vi "Keithley2612b_IV_vg_vd_reverse_sweeps_modified.vi"(3 "Error Query (False)":bool, 4 "Current Limit":dbl=1.0, 7 "Source Function (Current)":enum32{"Current", "Voltage"}(ring)=enum."Voltage", 8 "error in (no error)":errorcluster, 9 "Channel (Channel A)":T1, 10 "Node (0-64)":i8 min=0 max=64 step=1, 11 "VISA resource name":refnum<visa-resource-name>="Keithley_2612B") -> (0 "error out":errorcluster)   [LabVIEW 2016]
doc: "This example shows how to configure the source and take a measurement."
uses:
  <instrlib>/Keithley 2600 Series/Public/Channel.ctl
  <vilib>/express/express shared/transition.llb/Dynamic To Waveform Array.vi
  <vilib>/express/express signal manip/GetorSetDDTAttributes/Set DDT Attributes/SetT0.vi
  <vilib>/express/express shared/transition.llb/Waveform Array To Dynamic.vi
  <vilib>/express/express signal manip/GetorSetDDTAttributes/Set DDT Attributes/Set DDT Properties.xnode
  <instrlib>/Keithley 2600 Series/Keithley 2600 Series.lvlib
panel:
  out "Number for Vg":dbl
  out "Step Size ref":dbl
  out "XY Graph":cluster{dbl[], dbl[]}[](graph)
  out "Current Number":dbl
  in  "Reverse Sweep":bool
  in  "Current Limit 2":dbl=1.0
  in  "Source Function (Current) 2":enum32{"Current", "Voltage"}(ring)=enum."Voltage"
  in  "Channel (Channel A) 2":T1=enum."Channel B"
  out "Current Output 2":string
  in  "Delay (s) 2":dbl
  in  "Step Size 2":dbl=0.02
  in  "End Voltage 2":dbl=0.8
  in  "Start Voltage 2":dbl=-0.5
  out "Voltage Output 2":string
  out "Current Number Past 2":dbl
  out "Current Number Past":dbl
  out "Voltage Output":string
  out "Current Output":string
  in  "Delay (s)":dbl
  in  "Step Size":dbl=0.1
  in  "End Voltage":dbl=1.0
  in  "Start Voltage":dbl
  # "Gate Voltage"
  # "Drain Voltage"
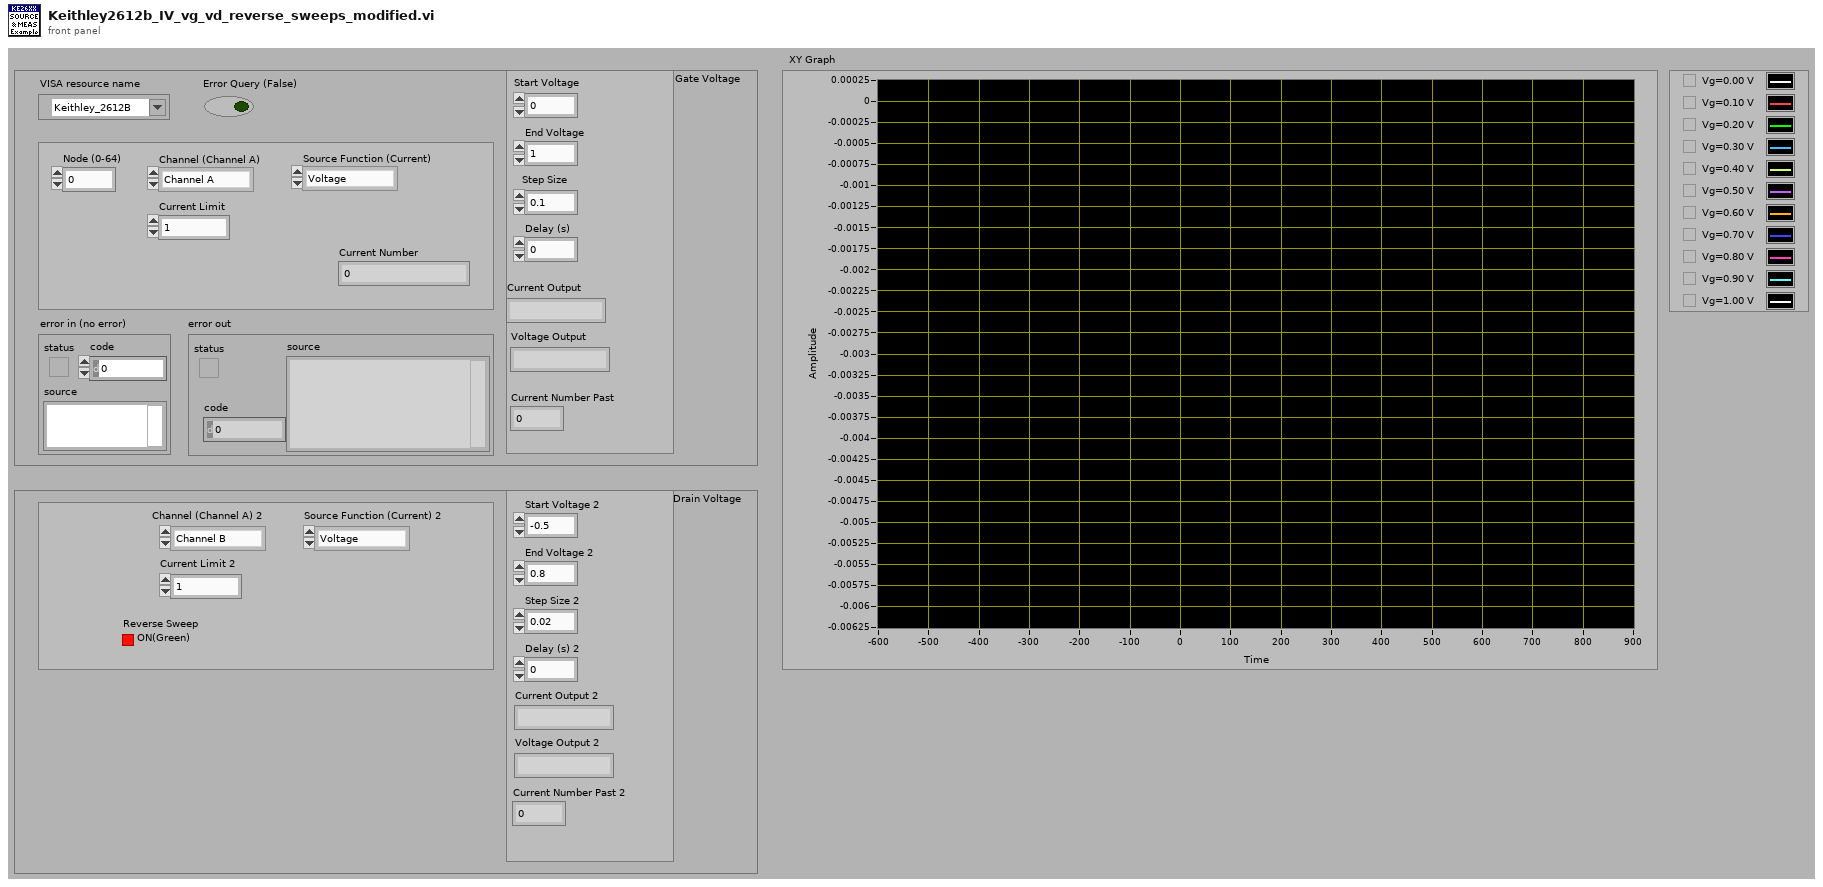
[diagram p1: front panel]
types:
  T1 = typedef "Keithley 2600 Series.lvlib/Channel.ctl" = enum32{"Channel A", "Channel B"}
  T2 = typedef "NI_Matrix.lvlib/RealMatrix.ctl" = dbl[][]
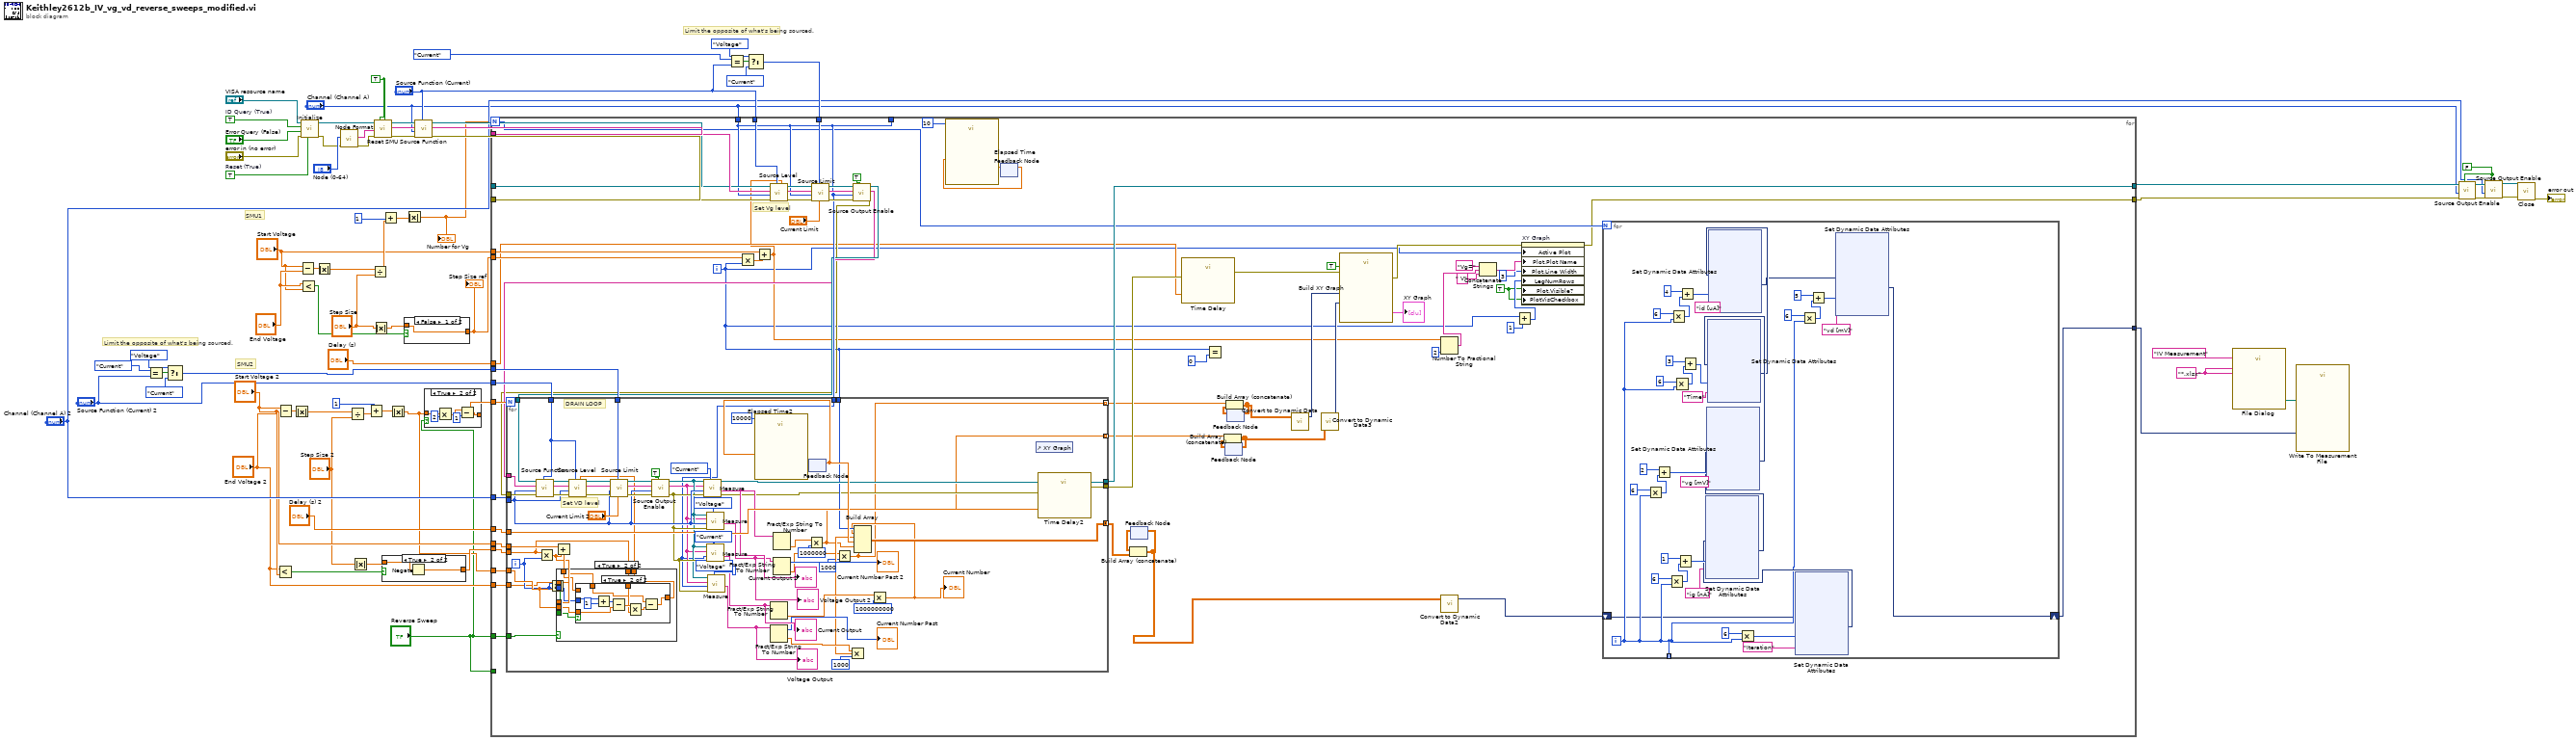
[diagram p0: block diagram]
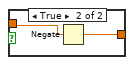
[diagram p3: hidden frame]
diagram:
  w29 = "*.xlsx"
  w40 = TRUE
  w24 = FALSE ("Output (Off)")
  w68 = TRUE  # Reset (True)
  w71 = TRUE  # ID Query (True)
  # "SMU2"
  # "SMU1"
  # "Limit the opposite of what's being sourced."
  # "Limit the opposite of what's being sourced."
  n1 = Equal?(x=enum32{"Current", "Voltage"}."Current", y="Source Function (Current) 2") -> (x = y?=w46:bool)
  n2 = Select(t=enum32{"Current", "Voltage"}."Voltage" ("x"), s=w46, f=enum32{"Current", "Voltage"}."Current") -> (s? t:f=w30:enum32{"Current", "Voltage"})
  n3 = Less?(x="End Voltage 2", y="Start Voltage 2") -> (x < y?=w20:bool)
  n4 = Subtract(x="Start Voltage 2", y="End Voltage 2") -> (x-y=w36:dbl)
  n5 = Absolute Value(x=w36) -> (abs(x)=w35:dbl)
  n6 = Subtract(x="Start Voltage", y="End Voltage") -> (x-y=w52:dbl)
  n7 = Less?(x="End Voltage", y="Start Voltage") -> (x < y?=w17:bool)
  n8 = call <instrlib>:"Initialize.vi"("Reset (True)"=w68, "error in (no error)"="error in (no error)", "Error Query (False)"="Error Query (False)", "ID Query (True)"=w71, "VISA resource name"="VISA resource name") -> ("error out"=w48:errorcluster, "VISA resource name out"=w41:refnum<visa-resource-name>)  [unwired: 1 in, 4 out]
  n9 = Absolute Value(x=w52) -> (abs(x)=w51:dbl)
  n10 = call <instrlib>:"Node Format.vi"("error in"=w48, "Node (0-64)"="Node (0-64)") -> ("error out"=w64:errorcluster, "Formatted Node"=w65:string)  [unwired: 8 out]
  n11 = Divide(x=w35, y="Step Size 2") -> (x/y=w33:dbl)
  n12 = Absolute Value(x="Step Size 2") -> (abs(x)=w14:dbl)
  n13 = Add(x=1, y=w33) -> (x+y=w12:dbl)
  n14 = Divide(x=w51, y="Step Size") -> (x/y=w49:dbl)
  n15 = Absolute Value(x="Step Size") -> (abs(x)=w8:dbl)
  n16 = call <instrlib>:"Reset SMU.vi"("SMU B (No)"=w40, "SMU A (No)"=w40, "error in (no error)"=w64, "Node In"=w65, "VISA resource name"=w41) -> ("error out"=w39:errorcluster, "Node Out"=w37:string, "VISA resource name out"=w38:refnum<visa-resource-name>)  [unwired: 4 out]
  n17 = Add(x=1, y=w49) -> (x+y=w11:dbl)
  n18 = case shown="True" w20 {
    tunnel: w14 -> [w72 w73]
    tunnel: [w72 w74] -> w15
    frame False {
    }
    frame True {
      n19 = Negate(x=w73) -> (-x=w74:dbl)
    }
  }
  n20 = Absolute Value(x=w12) -> (abs(x)=w5:dbl)
  n21 = case shown="False" w17 {
    tunnel: [w75 w77] -> w16
    tunnel: w8 -> [w75 w76]
    frame False {
    }
    frame True {
      n22 = Negate(x=w76) -> (-x=w77:dbl)
    }
  }
  "Step Size ref" <- w16
  n23 = Absolute Value(x=w11) -> (abs(x)=w10:dbl)
  "Number for Vg" <- w10
  n24 = call <instrlib>:"Source Function.vi"("Function (Current)"="Source Function (Current)", "error in (no error)"=w39, "Channel (Channel A)"="Channel (Channel A)", "Node In"=w37, "VISA resource name"=w38) -> ("error out"=w62:errorcluster, "Node Out"=w61:string, "VISA resource name out"=w60:refnum<visa-resource-name>)  [unwired: 4 out]
  n25 = case shown="True" "Reverse Sweep" {
    tunnel: w5 -> [w78 w83]
    tunnel: [w78 w81] -> w6
    frame False {
    }
    frame True {
      n26 = Multiply(x=w83, y=2) -> (x*y=w80:dbl)
      n27 = Subtract(x=w80, y=1) -> (x-y=w81:dbl)
    }
  }
  n28 = Equal?(x=enum32{"Current", "Voltage"}."Current", y="Source Function (Current)") -> (x = y?=w66:bool)
  n29 = Select(t=enum32{"Current", "Voltage"}."Voltage" ("x"), s=w66, f=enum32{"Current", "Voltage"}."Current") -> (s? t:f=w55:enum32{"Current", "Voltage"})
  n30 = for {
    N: w10 -> [w97]
    tunnel: w62 -> [w142]
    tunnel: w61 -> [w141]
    tunnel: w60 -> [w140]
    tunnel: "Channel (Channel A)" -> [w120]
    tunnel: "Source Function (Current)" -> [w138]
    tunnel: w16 -> [w113]
    tunnel: "Start Voltage" -> [w112]
    tunnel: w55 -> [w137]
    tunnel: [w131] -> w26
    tunnel: [w86] -> w1
    tunnel: "Delay (s)" -> [w110]
    tunnel: w15 -> [w133]
    tunnel: "Start Voltage 2" -> [w132]
    tunnel: "Delay (s) 2" -> [w130]
    tunnel: "Channel (Channel A) 2" -> [w129]
    tunnel: "Source Function (Current) 2" -> [w128]
    tunnel: w30 -> [w127]
    tunnel: [w120] -> _
    tunnel: w6 -> [w124]
    tunnel: "End Voltage 2" -> [w123]
    tunnel: "Reverse Sweep" -> [w122]
    tunnel: w5 -> [w121]
    tunnel: "Reverse Sweep" -> [_]
    tunnel: [w116] -> w3
    i -> [w84]
    w91 = TRUE
    # "Set Vg level"
    n31 = Multiply(x=w113, y=w84) -> (x*y=w139:dbl)
    n32 = Add(x=w112, y=w139) -> (x+y=w85:dbl)
    n33 = call <instrlib>:"Source Level.vi"("Level (0.000)"=w85, "Function (Current)"=w138, "error in (no error)"=w142, "Channel (Channel A)"=w120, "Node In"=w141, "VISA resource name"=w140) -> ("error out"=w143:errorcluster, "Node Out"=w148:string, "VISA resource name out"=w144:refnum<visa-resource-name>)  [unwired: 3 out]
    n34 = call <instrlib>:"Source Limit.vi"("Limit (0.000)"="Current Limit", "Function (Current)"=w137, "error in (no error)"=w143, "Channel (Channel A)"=w120, "Node In"=w148, "VISA resource name"=w144) -> ("error out"=w146:errorcluster, "Node Out"=w149:string, "VISA resource name out"=w145:refnum<visa-resource-name>)  [unwired: 3 out]
    n35 = call <instrlib>:"Source Output Enable.vi"("Output (Off)"=TRUE, "error in (no error)"=w146, "Channel (Channel A)"=w120, "Node In"=w149, "VISA resource name"=w145) -> ("error out"=w117:errorcluster, "Node Out"=w118:string, "VISA resource name out"=w119:refnum<visa-resource-name>)  [unwired: 4 out]
    n36 = for {
      N: w124 -> [_]
      tunnel: w118 -> [w305]
      tunnel: w133 -> [w291]
      tunnel: w132 -> [w318]
      tunnel: w127 -> [w317]
      tunnel: [w309] -> w131
      tunnel: [w316] -> w111
      tunnel: w117 -> [w306]
      tunnel: w119 -> [w304]
      tunnel: w130 -> [w308]
      tunnel: w129 -> [w299]
      tunnel: w128 -> [w301]
      tunnel: [w300] -> w125 mode=concatenating
      tunnel: w84 -> [w277]
      tunnel: w123 -> [w290]
      tunnel: w122 -> [w298]
      tunnel: w121 -> [w294]
      tunnel: w120 -> [w284]
      tunnel: [w266] -> w103 mode=indexing
      tunnel: [w265] -> w108 mode=indexing
      i -> [w292]
      # "Set VD level"
      # "DRAIN LOOP"
      n37 = call <instrlib>:"Source Function.vi"("Function (Current)"=w301, "error in (no error)"=w306, "Channel (Channel A)"=w299, "Node In"=w305, "VISA resource name"=w304) -> ("error out"=w307:errorcluster, "Node Out"=w303:string, "VISA resource name out"=w302:refnum<visa-resource-name>)  [unwired: 4 out]
      n38 = Multiply(x=w291, y=w292) -> (x*y=w293:dbl)
      n39 = Greater Or Equal?(x=w292, y=w294) -> (x >= y?=w295:bool)
      n40 = Add(x=w318, y=w293) -> (x+y=w297:dbl)
      n41 = case shown="True" w298 {
        tunnel: w295 -> [_ w334]
        tunnel: w297 -> [w327 w333]
        tunnel: [w327 w332] -> w296
        tunnel: w294 -> [_ w331]
        tunnel: w293 -> [_ _]
        tunnel: w292 -> [_ w330]
        tunnel: w291 -> [_ w329]
        tunnel: w290 -> [_ w328]
        frame False {
        }
        frame True {
          n42 = case shown="True" w334 {
            tunnel: w333 -> [w335 _]
            tunnel: [w335 w336] -> w332
            tunnel: w331 -> [_ w343]
            tunnel: w330 -> [_ w342]
            tunnel: w329 -> [_ w339]
            tunnel: w328 -> [_ w337]
            frame False {
            }
            frame True {
              n43 = Add(x=w342, y=1) -> (x+y=w344:i32)
              n44 = Subtract(x=w344, y=w343) -> (x-y=w340:dbl)
              n45 = Multiply(x=w340, y=w339) -> (x*y=w338:dbl)
              n46 = Subtract(x=w337, y=w338) -> (x-y=w336:dbl)
            }
          }
        }
      }
      n47 = call <instrlib>:"Source Level.vi"("Level (0.000)"=w296, "Function (Current)"=w301, "error in (no error)"=w307, "Channel (Channel A)"=w299, "Node In"=w303, "VISA resource name"=w302) -> ("error out"=w319:errorcluster, "Node Out"=w324:string, "VISA resource name out"=w320:refnum<visa-resource-name>)  [unwired: 3 out]
      n48 = call <instrlib>:"Source Limit.vi"("Limit (0.000)"="Current Limit 2", "Function (Current)"=w317, "error in (no error)"=w319, "Channel (Channel A)"=w299, "Node In"=w324, "VISA resource name"=w320) -> ("error out"=w322:errorcluster, "Node Out"=w325:string, "VISA resource name out"=w321:refnum<visa-resource-name>)  [unwired: 3 out]
      n49 = call <instrlib>:"Source Output Enable.vi"("Output (Off)"=TRUE, "error in (no error)"=w322, "Channel (Channel A)"=w299, "Node In"=w325, "VISA resource name"=w321) -> ("error out"=w287:errorcluster, "Node Out"=w285:string, "VISA resource name out"=w286:refnum<visa-resource-name>)  [unwired: 4 out]
      n50 = call <instrlib>:"Measure.vi"("Function (Current)"=enum32{"Current", "Voltage"}."Current" ("x"), "error in (no error)"=w287, "Channel (Channel A)"=w299, "Node In"=w285, "VISA resource name"=w286) -> ("error out"=w267:errorcluster, "Output"=w280:string, "VISA resource name out"=w309:refnum<visa-resource-name>)  [unwired: 2 in, 2 out]
      "Current Output 2" <- w280
      n51 = call <instrlib>:"Measure.vi"("Function (Current)"=enum32{"Current", "Voltage"}."Voltage" ("x"), "error in (no error)"=w287, "Channel (Channel A)"=w299, "Node In"=w285, "VISA resource name"=w286) -> ("Output"=w279:string)  [unwired: 2 in, 4 out]
      "Voltage Output 2" <- w279
      n52 = call <instrlib>:"Measure.vi"("Function (Current)"=enum32{"Current", "Voltage"}."Current" ("x"), "error in (no error)"=w287, "Channel (Channel A)"=w284, "Node In"=w285, "VISA resource name"=w286) -> ("Output"=w283:string)  [unwired: 2 in, 4 out]
      "Current Output" <- w283
      n53 = call <instrlib>:"Measure.vi"("Function (Current)"=enum32{"Current", "Voltage"}."Voltage" ("x"), "error in (no error)"=w287, "Channel (Channel A)"=w284, "Node In"=w285, "VISA resource name"=w286) -> ("Output"=w282:string)  [unwired: 2 in, 4 out]
      "Voltage Output" <- w282
      n54 = Fract/Exp String To Number(string=w282) -> (offset past number=→"Current Number Past":i32, number=w271:dbl)  [unwired: 3 in]
      n55 = Fract/Exp String To Number(string=w283) -> (number=w273:dbl)  [unwired: 3 in, 1 out]
      n56 = Fract/Exp String To Number(string=w279) -> (offset past number=→"Current Number Past 2":i32, number=w268:dbl)  [unwired: 3 in]
      n57 = Fract/Exp String To Number(string=w280) -> (number=w274:dbl)  [unwired: 3 in, 1 out]
      n58 = Multiply(x=w274, y=1000000) -> (x*y=w266:dbl)
      n59 = feedback #1() -> (w310:dbl)  [unwired: 1 in]
      n60 = call "Elapsed Time2"("Time Target (s)"=10000, "Set Start Time (s)"=w310) -> ("Elapsed Time (s)"=w313:dbl)  [unwired: 10 in, 7 out]
      n61 = feedback-in #1(w313) -> ()
      n62 = Multiply(x=w268, y=1000) -> (x*y=w265:dbl)
      n63 = Multiply(x=w271, y=1000) -> (x*y=w270:dbl)
      n64 = Multiply(x=w273, y=1000000000) -> (x*y=w276:dbl)
      "Current Number" <- w276
      n65 = Build Array(w277, w276, w270, w310, w266, w265) -> (w300:T2)
      n66 = control-ref of="XY Graph"() -> ()  [unwired: 1 out]
      n67 = call "Time Delay2"("error in (no error)"=w267, "Delay Time (s)"=w308) -> ("error out"=w316:errorcluster)  [unwired: 9 in]
    }
    n68 = feedback #2() -> (w134:dbl)  [unwired: 1 in]
    n69 = call "Elapsed Time"("Time Target (s)"=10, "Set Start Time (s)"=w134) -> ("Elapsed Time (s)"=w136:dbl)  [unwired: 10 in, 7 out]
    n70 = feedback-in #2(w136) -> ()
    n71 = feedback #3() -> (w126:T2)  [unwired: 1 in]
    n72 = Build Array (concatenate)(w126, w125) -> (w115:T2)
    n73 = feedback-in #3(w115) -> ()
    n74 = call "Time Delay"("error in (no error)"=w111, "Delay Time (s)"=w110) -> ("error out"=w107:errorcluster)  [unwired: 9 in]
    n75 = Equal?(x=w84, y=0) -> ()  [unwired: 1 out]
    n76 = feedback #4() -> (w104:dbl[][])  [unwired: 1 in]
    n77 = Build Array (concatenate)(w103, w104) -> (w101:dbl[][])
    n78 = feedback-in #4(w101) -> ()
    n79 = feedback #5() -> (w106:dbl[][])  [unwired: 1 in]
    n80 = Build Array (concatenate)(w108, w106) -> (w105:dbl[][])
    n81 = feedback-in #5(w105) -> ()
    n82 = call "Convert to Dynamic Data"("2D Array"=w105) -> ("Dynamic Data Type"=w102:dynamicdata)  [unwired: 3 in]
    n83 = call "Convert to Dynamic Data3"("2D Array"=w101) -> ("Dynamic Data Type"=w100:dynamicdata)  [unwired: 3 in]
    n84 = call "Build XY Graph"("error in (no error)"=w107, "Reset"=TRUE, "Y Input"=w100, "X Input"=w102) -> ("error out"=w87:errorcluster, "XY Graph"=→"XY Graph":cluster{"X":dbl[], "Y":dbl[]}[])  [unwired: 6 in]
    n85 = Number To Fractional String(number=w85, precision (6)=2) -> (F-format string=w94:string)  [unwired: 2 in]
    n86 = call "Convert to Dynamic Data2"("2D Array"=w115) -> ("Dynamic Data Type"=w114:dynamicdata)  [unwired: 3 in]
    n87 = Concatenate Strings("Vg=", w94, " V") -> (w90:string)
    n88 = Add(x=w84, y=1) -> (x+y=w92:i32)
    n89 = property on="XY Graph" class="XYGraph (strict)"(error in=w87, "Active Plot"=w84, "Plot.Plot Name"=w90, "Plot.Line Width"=3, "LegNumRows"=w92, "Plot.Visible?"=w91, "PlotVisCheckbox"=w91) -> (error out=w86:errorcluster)  [unwired: 1 in, 1 out]
    n90 = for {
      N: w97 -> [_]
      shift-right: [w151] -> w116
      shift-left: w114 -> [w152]
      tunnel: [w153] -> _ mode=indexing
      i -> [w153]
      n91 = Multiply(x=6, y=w153) -> (x*y=w179:i32)
      n92 = Add(x=2, y=w179) -> (x+y=w172:i32)
      n93 = Multiply(x=6, y=w153) -> (x*y=w182:i32)
      n94 = Multiply(x=6, y=w153) -> (x*y=w173:i32)
      n95 = Multiply(x=6, y=w153) -> (x*y=w176:i32)
      n96 = Add(x=1, y=w182) -> (x+y=w168:i32)
      n97 = Add(x=4, y=w173) -> (x+y=w167:i32)
      n98 = Add(x=3, y=w176) -> (x+y=w154:i32)
      n99 = Multiply(x=6, y=w153) -> (x*y=w185:i32)
      n100 = xnode "Set Dynamic Data Attributes"("Signals In"=w152, "Signal Index"=w185, "Signal Name"="Iteration") -> ("Signals Out"=w165:dynamicdata)  [unwired: 1 in, 1 out]
      n101 = xnode "Set Dynamic Data Attributes"("Signals In"=w165, "Signal Index"=w168, "Signal Name"="ig [nA]") -> ("Signals Out"=w164:dynamicdata)  [unwired: 1 in, 1 out]
      n102 = xnode "Set Dynamic Data Attributes"("Signals In"=w164, "Signal Index"=w172, "Signal Name"="vg [mV]") -> ("Signals Out"=w163:dynamicdata)  [unwired: 1 in, 1 out]
      n103 = xnode "Set Dynamic Data Attributes"("Signals In"=w163, "Signal Index"=w154, "Signal Name"="Time") -> ("Signals Out"=w162:dynamicdata)  [unwired: 1 in, 1 out]
      n104 = xnode "Set Dynamic Data Attributes"("Signals In"=w162, "Signal Index"=w167, "Signal Name"="id [uA]") -> ("Signals Out"=w161:dynamicdata)  [unwired: 1 in, 1 out]
      n105 = Multiply(x=6, y=w153) -> (x*y=w169:i32)
      n106 = Add(x=5, y=w169) -> (x+y=w166:i32)
      n107 = xnode "Set Dynamic Data Attributes"("Signals In"=w161, "Signal Index"=w166, "Signal Name"="vd [mV]") -> ("Signals Out"=w151:dynamicdata)  [unwired: 1 in, 1 out]
    }
  }
  n108 = call "File Dialog"("default name"="IV Measurement", "pattern (all files)"=w29, "pattern label"=w29) -> ("selected path"=w22:path)  [unwired: 9 in, 3 out]
  n109 = call "Write To Measurement File"("Signals"=w3, "Filename"=w22) -> ()  [unwired: 15 in, 3 out]
  n110 = call <instrlib>:"Source Output Enable.vi"("Output (Off)"=w24, "error in (no error)"=w1, "Channel (Channel A)"="Channel (Channel A)", "VISA resource name"=w26) -> ("error out"=w25:errorcluster, "VISA resource name out"=w27:refnum<visa-resource-name>)  [unwired: 1 in, 5 out]
  n111 = call <instrlib>:"Source Output Enable.vi"("Output (Off)"=w24, "error in (no error)"=w25, "Channel (Channel A)"="Channel (Channel A) 2", "VISA resource name"=w27) -> ("error out"=w56:errorcluster, "VISA resource name out"=w57:refnum<visa-resource-name>)  [unwired: 1 in, 5 out]
  n112 = call <instrlib>:"Close.vi"("error in (no error)"=w56, "VISA resource name"=w57) -> ("error out"=→"error out":errorcluster)  [unwired: 9 out]
